vi "AB_HasGInterface.vi"(8 "error in (no error)":errorcluster, 10 "itemID":string, 11 "Project Refnum":refnum<vi>) -> (0 "error out":errorcluster, 3 "Has G Interface":bool)   [LabVIEW 2020]
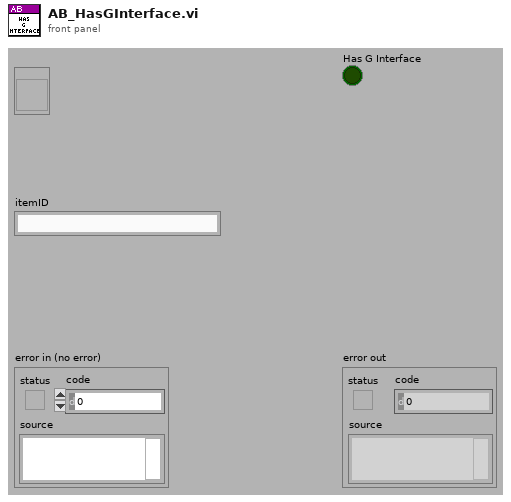
[diagram p1: front panel]
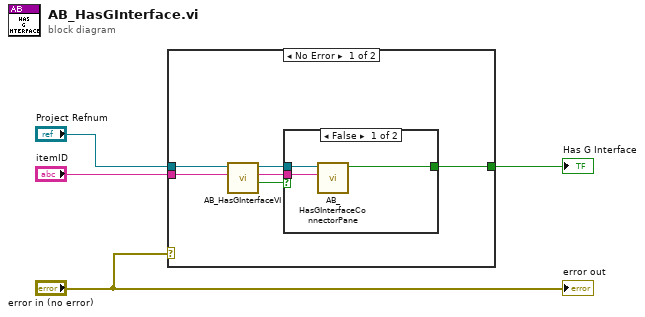
[diagram p0: block diagram]
diagram:
  n1 = case shown="No Error" "error in (no error)" {
    tunnel: "itemID" -> [w8 _]
    tunnel: "Project Refnum" -> [w9 _]
    tunnel: [w10 _] -> w2
    frame No Error {
      n2 = call <vilib>:"AB_HasGInterfaceVI.vi"("itemID"=w8, "Project Refnum"=w9) -> ("Has G Interface"=w7:bool, "itemID dup"=w5:string, "Project Refnum dup"=w6:refnum<vi>)  [unwired: 6 in, 1 out]
      n3 = case shown="False" w7 {
        selector: w7 -> [_ w14]
        tunnel: [w12 w14] -> w10
        tunnel: w6 -> [w13 _]
        tunnel: w5 -> [w11 _]
        frame False {
          n4 = call <vilib>:"AB_HasGInterfaceConnectorPane.vi"("itemID"=w11, "Project Refnum"=w13) -> ("Has G Interface"=w12:bool)  [unwired: 8 in, 1 out]
        }
        frame True {
        }
      }
    }
    frame Error {
    }
  }
  "Has G Interface" <- w2
  "error out" <- "error in (no error)"
